vi "I2C LCD Raw ADC.vi"() -> ()   [LabVIEW 2020, in "CTI-Scratchpad.lvlib"]
uses:
  CTI-Scratchpad.lvlib
  CTI-Visa-DeviceLib/LCD-I2C/LCD-I2C.lvclass
  CTI-Visa-DeviceLib/LCD-I2C/Position.ctl
  <vilib>/ptbypt/NI_PtbyPt.lvlib
  CTI/VisaComms/VisaComms.lvclass
  CTI/Session/Session.lvclass
  CTI/AI/AI.lvclass
  CTI-Visa-DeviceLib/LCD-I2C/LCD Size.ctl
  CTI-Visa/I2C Options.ctl
  CTI-Visa/CTI-Visa.lvlib
  CTI/I2C Address.ctl
  CTI/CTI.lvlib
  CTI/ADC Number.ctl
panel:
  out "Rate":dbl format="%0.2f"
  out "Value":u16
  in  "ADC":T1
  in  "Address":T2=39 format="%02x"
  in  "I2C Options":T3={"Bus"=0, "Baud"=400000, "SCL GPIO"=16, "SDA GPIO"=17}
  in  "LCD Size":T4={"Rows"=2, "Cols"=16}
  in  "stop":bool
  out "error out":errorcluster
  in  "Port":refnum<visa-resource-name>="COM4"
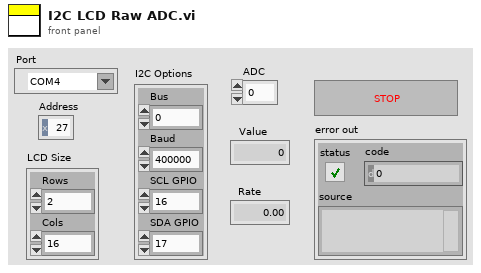
[diagram p1: front panel]
types:
  T1 = typedef "CTI.lvlib/ADC Number.ctl" = i8
  T2 = typedef "CTI.lvlib/I2C Address.ctl" = u8
  T3 = typedef "CTI-Visa.lvlib/I2C Options.ctl" = cluster{"Bus":u8, "Baud":u32, "SCL GPIO":i32, "SDA GPIO":i32}
  T4 = typedef "CTI-Visa-DeviceLib.lvlib/LCD-I2C.lvclass/LCD Size.ctl" = cluster{"Rows":u8, "Cols":u8}
  T5 = typedef "CTI-Visa-DeviceLib.lvlib/LCD-I2C.lvclass/Position.ctl" = cluster{"Row":u8, "Col":u8}
  T6 = typedef "CTI.lvlib/Raw ADC.ctl" = u16
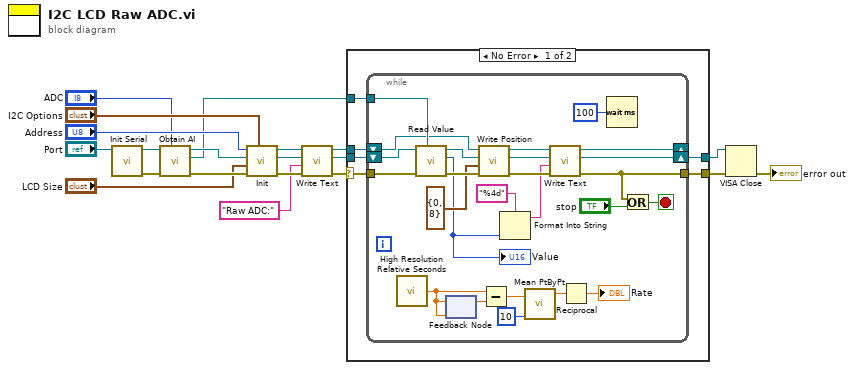
[diagram p0: block diagram]
diagram:
  n1 = call "Init Serial.vi"("VISA resource name in"="Port") -> ("error out"=w11:errorcluster, "Session"=w12:refnum<class "Session.lvclass">)  [unwired: 9 in]
  n2 = call "Obtain AI.vi"("ADC #"="ADC", "error in (no error)"=w11, "Session in"=w12) -> ("error out"=w20:errorcluster, "AI"=w1:refnum<class "AI.lvclass">, "Session out"=w4:refnum<class "Session.lvclass">)  [unwired: 6 in]
  n3 = call "Init.vi"("I2C Options"="I2C Options", "error in (no error)"=w20, "LCD Size"="LCD Size", "VISA resource name in"=w4, "Address"="Address") -> ("error out"=w15:errorcluster, "VISA resource name"=w7:refnum<visa-resource-name>, "LCD-I2C out"=w9:refnum<class "LCD-I2C.lvclass">)  [unwired: 4 in]
  n4 = call "Write Text.vi"("error in (no error)"=w15, "Text"="Raw ADC:", "VISA resource name in"=w7, "LCD-I2C in"=w9) -> ("error out"=w10:errorcluster, "VISA resource name"=w6:refnum<visa-resource-name>, "LCD-I2C out"=w8:refnum<class "LCD-I2C.lvclass">)  [unwired: 5 in]
  n5 = case shown="No Error" w10 {
    selector: w10 -> [w24 w53]
    tunnel: w6 -> [w25 w52]
    tunnel: w8 -> [w26 _]
    tunnel: [w21 w53] -> w14
    tunnel: [w23 w52] -> w13
    tunnel: w1 -> [w22 _]
    frame No Error {
      n6 = while {
        shift-right: [w37] -> _
        shift-left: w26 -> [w47]
        shift-right: [w38] -> w23
        shift-left: w25 -> [w50]
        tunnel: w24 -> [w49]
        tunnel: w22 -> [w48]
        tunnel: [w39] -> w21
        stop <- w51 stop-if-true
        n7 = call <vilib>:"High Resolution Relative Seconds.vi"() -> ("relative seconds"=w32:dbl)
        n8 = call "Read Value.vi"("AnalogIn"=w48, "error in (no error)"=w49, "Session In"=w50) -> ("error out"=w45:errorcluster, "Value"=w35:T6, "Session Out"=w46:refnum<class "Session.lvclass">)  [unwired: 6 in]
        "Value" <- w35
        n9 = feedback-in #1(w32) -> ()
        n10 = feedback #1(w32) -> (w31:dbl)
        n11 = call "Write Position.vi"("error in (no error)"=w45, "Position"=T5 {"Row"=0, "Col"=8}, "VISA resource name in"=w46, "LCD-I2C in"=w47) -> ("error out"=w40:errorcluster, "VISA resource name"=w41:refnum<visa-resource-name>, "LCD-I2C out"=w42:refnum<class "LCD-I2C.lvclass">)  [unwired: 5 in]
        n12 = Subtract(x=w32, y=w31) -> (x-y=w30:dbl)
        n13 = Format Into String(format string="%4d", w35) -> (resulting string=w34:string)  [unwired: 2 in, 1 out]
        n14 = call <vilib>:"Mean PtByPt.vi"("x"=w30, "sample length"=10) -> ("mean"=w28:dbl)  [unwired: 2 in, 1 out]
        n15 = call "Write Text.vi"("error in (no error)"=w40, "Text"=w34, "VISA resource name in"=w41, "LCD-I2C in"=w42) -> ("error out"=w39:errorcluster, "VISA resource name"=w38:refnum<visa-resource-name>, "LCD-I2C out"=w37:refnum<class "LCD-I2C.lvclass">)  [unwired: 5 in]
        n16 = Reciprocal(x=w28) -> (1/x=→"Rate":dbl)
        n17 = Wait (ms)(milliseconds to wait=u32 100) -> ()  [unwired: 1 out]
        n18 = Or(x=w39, y="stop") -> (x .or. y?=w51:bool)
      }
    }
    frame Error {
    }
  }
  n19 = VISA Close(VISA resource name=w13, error in (no error)=w14) -> (error out=→"error out":errorcluster)
